vi "x502_out_cfg.vi"(3 "error in (no error)":errorcluster, 4 "FoutCfg":dbl=1000000.0, 5 "x502 in":refnum<k24>) -> (0 "error out":errorcluster, 1 "Fout":dbl, 2 "x502 out":refnum<k24>)   [LabVIEW 2010]
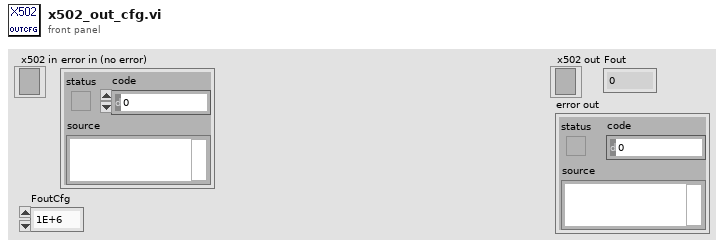
[diagram p1: front panel]
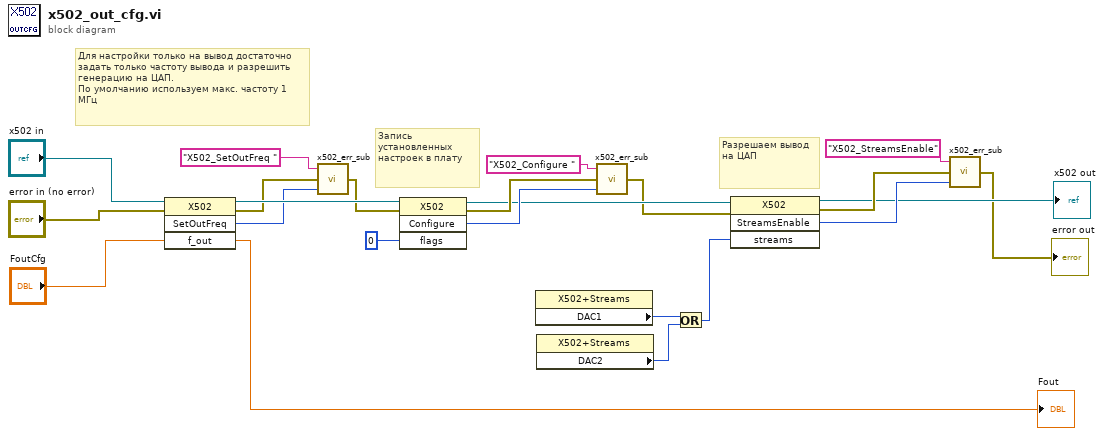
[diagram p0: block diagram]
diagram:
  # "Для настройки только на вывод достаточно задать только частоту вывода и разрешить генерацию на ЦАП.\nПо умолчанию используем макс. частоту 1 МГц"
  # "Разрешаем вывод на ЦАП"
  # "Запись установленных настроек в плату"
  n1 = invoke class="X502" method="SetOutFreq"(reference="x502 in", error in="error in (no error)", "f_out"="FoutCfg") -> (reference out=w14:refnum<k24>, error out=w8:errorcluster, "SetOutFreq"=w7:i32, "f_out"=→"Fout":dbl)  [unwired: 1 in]
  n2 = call "x502_err_sub.vi"("Error code"=w7, "error in (no error)"=w8, "Error descr"="X502_SetOutFreq ") -> ("error out"=w6:errorcluster)
  n3 = invoke class="X502" method="Configure"(reference=w14, error in=w6, "flags"=0) -> (reference out=w16:refnum<k24>, error out=w22:errorcluster, "Configure"=w21:i32)  [unwired: 1 in, 1 out]
  n4 = property class="X502+Streams"() -> ("DAC1"=w18:u32)  [unwired: 2 in, 2 out]
  n5 = property class="X502+Streams"() -> ("DAC2"=w19:u32)  [unwired: 2 in, 2 out]
  n6 = call "x502_err_sub.vi"("Error code"=w21, "error in (no error)"=w22, "Error descr"="X502_Configure ") -> ("error out"=w15:errorcluster)
  n7 = Or(x=w18, y=w19) -> (x .or. y?=w17:u32)
  n8 = invoke class="X502" method="StreamsEnable"(reference=w16, error in=w15, "streams"=w17) -> (reference out=→"x502 out":refnum<k24>, error out=w4:errorcluster, "StreamsEnable"=w3:i32)  [unwired: 1 in, 1 out]
  n9 = call "x502_err_sub.vi"("Error code"=w3, "error in (no error)"=w4, "Error descr"="X502_StreamsEnable") -> ("error out"=→"error out":errorcluster)
